vi "Set Tree Symbols.vi"(7 "Path to PNG lib":path, 8 "error in (no error)":errorcluster, 10 "Index and Image":cluster{"DataType":T1, "FileName":string}[](array[cluster]), 11 "TreeControl in":refnum<vi>) -> (0 "error out":errorcluster)   [LabVIEW 2017, in "Shared Variables CD 2.0 Configuration.lvlib"]
uses:
  Shared Variables CD 2.0 Configuration.lvlib
  <vilib>/Utility/Data Type/Type Definitions/Data Type.ctl
  <vilib>/Utility/Data Type/NI_Data Type.lvlib
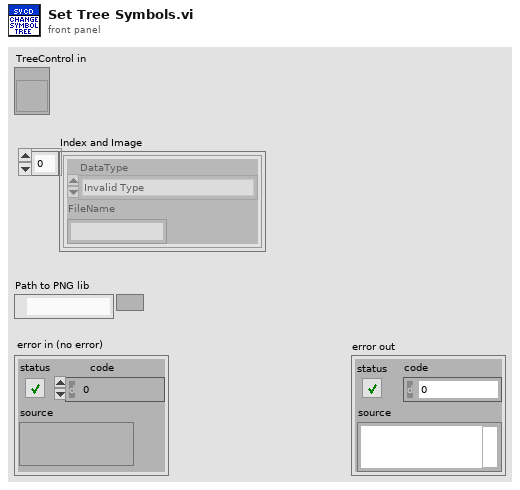
[diagram p1: front panel]
types:
  T1 = typedef "NI_Data Type.lvlib/Data Type.ctl" = enum8{"Invalid Type", "Void", "I8", "I16", "I32", "I64", "U8", "U16", "U32", "U64", "Single Float", "Double Float", "Extended Float", "Single Complex", "Double Complex", "Extended Complex", "Enum U8", "Enum U16", "Enum U32", "Enum U64", "Single Float With Unit", "Double Float With Unit", "Extended Float With Unit", "Single Complex with Unit", "Double Complex with Unit", "Extended Complex with Unit", "Boolean", "String", "Path", "Picture", "Tag", "Array", "Cluster", "Variant", "LV Variant", "Waveform", "Timestamp", "Digital Waveform", "Digital Data", "ExpressData", "Refnum", "External Data", "VI", "Poly VI", "LabVIEW Class Instance", "Fixed Point"}
  T2 = typedef "imagedata.ctl" = cluster{"image type":i32, "image depth":i32, "image":u8[], "mask":u8[], "colors":u32[], "Rectangle":cluster{"left":i16, "top":i16, "right":i16, "bottom":i16}}
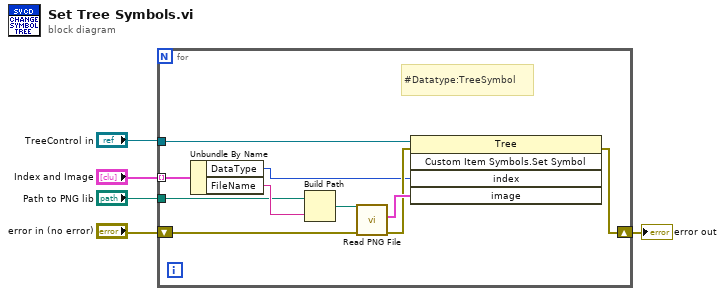
[diagram p0: block diagram]
diagram:
  n1 = for {
    tunnel: "TreeControl in" -> [w15]
    tunnel: "Index and Image" -> [w13] mode=indexing
    shift-right: [w10] -> w2
    shift-left: "error in (no error)" -> [w11]
    tunnel: "Path to PNG lib" -> [w8]
    # "#Datatype:TreeSymbol"
    n2 = Unbundle By Name(w13) -> ("DataType"=w6:T1, "FileName"=w9:string)
    n3 = Build Path(base path=w8, name or relative path=w9) -> (appended path=w7:path)
    n4 = call <vilib>:"Read PNG File.vi"("error in (no error)"=w11, "path to PNG file"=w7) -> ("error out"=w12:errorcluster, "image data"=w14:T2)  [unwired: 7 in, 1 out]
    n5 = invoke class="Tree" method="Custom Item Symbols.Set Symbol"(reference=w15, error in=w12, "index"=w6, "image"=w14) -> (error out=w10:errorcluster)  [unwired: 1 in, 4 out]
  }
  "error out" <- w2
